vi "Move Head.vi"(7 "XYGraph in":refnum<vi>, 10 "Direction":string, 11 "Rope in":cluster{"x":i64, "y":i64}[](array[cluster])) -> (3 "Rope out":cluster{"x":i64, "y":i64}[](array[cluster]), 5 "XY Graph out":refnum<vi>)   [LabVIEW 2021, in "d9.lvlib"]
uses:
  d9.lvlib
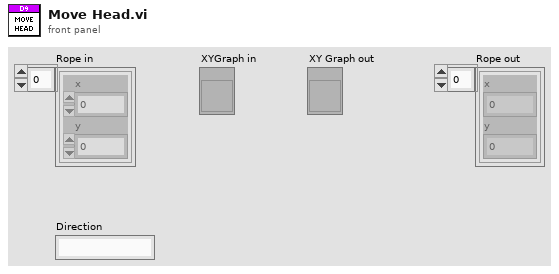
[diagram p1: front panel]
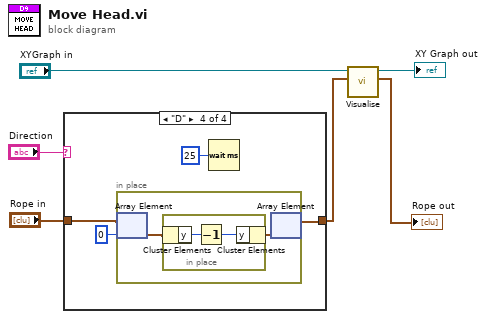
[diagram p0: block diagram]
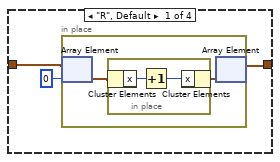
[diagram p2: hidden frame]
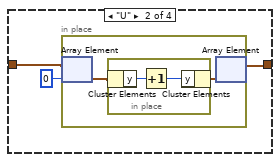
[diagram p3: hidden frame]
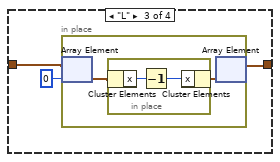
[diagram p4: hidden frame]
diagram:
  n1 = case shown="\"D\"" "Direction" {
    tunnel: "Rope in" -> [w9 w16 w23 w31]
    tunnel: [w7 w14 w21 w29] -> w2
    frame "R", Default {
      n2 = in-place {
        n3 = in-place-array #1(w9, 0) -> (w11:cluster{"x":i64, "y":i64})
        n4 = in-place {
          n5 = in-place-cluster #2(w11) -> ("x"=w13:i64)
          n6 = Increment(x=w13) -> (x+1=w12:i64)
          n7 = in-place-cluster #2("x"=w12) -> (w10:cluster{"x":i64, "y":i64})
        }
        n8 = in-place-array #1(w10) -> (w7:cluster{"x":i64, "y":i64}[])  [unwired: 1 out]
      }
    }
    frame "U" {
      n9 = in-place {
        n10 = in-place-array #3(w16, 0) -> (w18:cluster{"x":i64, "y":i64})
        n11 = in-place {
          n12 = in-place-cluster #4(w18) -> ("y"=w20:i64)
          n13 = Increment(x=w20) -> (x+1=w19:i64)
          n14 = in-place-cluster #4("y"=w19) -> (w17:cluster{"x":i64, "y":i64})
        }
        n15 = in-place-array #3(w17) -> (w14:cluster{"x":i64, "y":i64}[])  [unwired: 1 out]
      }
    }
    frame "L" {
      n16 = in-place {
        n17 = in-place-array #5(w23, 0) -> (w25:cluster{"x":i64, "y":i64})
        n18 = in-place {
          n19 = in-place-cluster #6(w25) -> ("x"=w27:i64)
          n20 = Decrement(x=w27) -> (x-1=w26:i64)
          n21 = in-place-cluster #6("x"=w26) -> (w24:cluster{"x":i64, "y":i64})
        }
        n22 = in-place-array #5(w24) -> (w21:cluster{"x":i64, "y":i64}[])  [unwired: 1 out]
      }
    }
    frame "D" {
      n23 = in-place {
        n24 = in-place-array #7(w31, 0) -> (w33:cluster{"x":i64, "y":i64})
        n25 = in-place {
          n26 = in-place-cluster #8(w33) -> ("y"=w35:i64)
          n27 = Decrement(x=w35) -> (x-1=w34:i64)
          n28 = in-place-cluster #8("y"=w34) -> (w32:cluster{"x":i64, "y":i64})
        }
        n29 = in-place-array #7(w32) -> (w29:cluster{"x":i64, "y":i64}[])  [unwired: 1 out]
      }
      n30 = Wait (ms)(milliseconds to wait=u32 25) -> ()  [unwired: 1 out]
    }
  }
  n31 = call "Visualise.vi"("Rope in"=w2, "XYGraph in"="XYGraph in") -> ("Rope out"=→"Rope out":cluster{"x":i64, "y":i64}[], "XY Graph out"=→"XY Graph out":refnum<vi>)  [unwired: 8 in]
